vi "Get Channel Group.vi"(8 "error in (no error)":errorcluster, 9 "ChanGroup":i32, 11 "TimingGrp in":refnum<class "TimingGrp.lvclass">) -> (0 "error out":errorcluster, 3 "Chan Gropu":refnum<class "ChanGrp.lvclass">)   [LabVIEW 2012, in "Configuration Grandmaster.lvlib" / "TimingGrp.lvclass"]
uses:
  TimingGrp.lvclass
  Class Chan Group/ChanGrp.lvclass
  TimingGrp.lvclass/TimingGrp.ctl
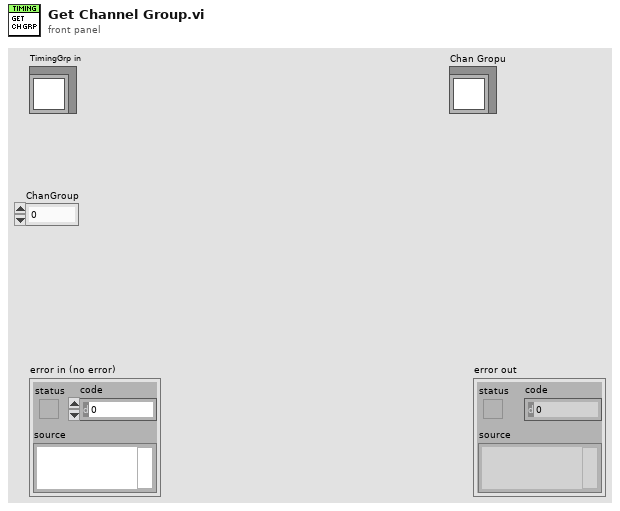
[diagram p1: front panel]
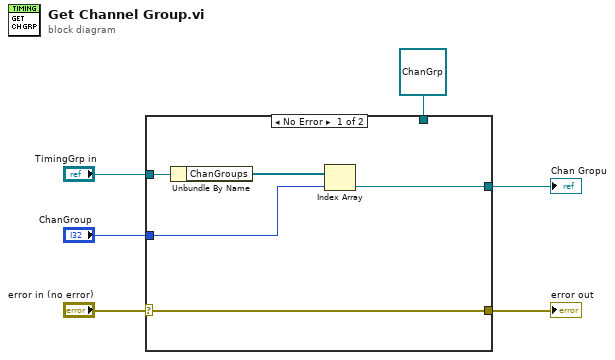
[diagram p0: block diagram]
diagram:
  n1 = case shown="No Error" "error in (no error)" {
    selector: "error in (no error)" -> [w11 w13]
    tunnel: [w11 w13] -> w5
    tunnel: "TimingGrp in" -> [w10 _]
    tunnel: "ChanGroup" -> [w8 _]
    tunnel: [w7 w12] -> w2
    tunnel: refnum<class "ChanGrp.lvclass"> refnum ("GroupChans.lvclass") -> [_ w12]
    frame No Error {
      n2 = Unbundle By Name(w10) -> ("ChanGroups"=w9:refnum<class "ChanGrp.lvclass">[])
      n3 = Index Array(array=w9, index=w8) -> (element=w7:refnum<class "ChanGrp.lvclass">)
    }
    frame Error {
    }
  }
  "error out" <- w5
  "Chan Gropu" <- w2
